vi "实时数据发送 (子VI).vi"(11 "数值":i32) -> ()   [LabVIEW 2016, in "数据传输系统.lvlib"]
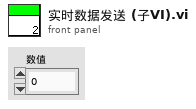
[diagram p1: front panel]
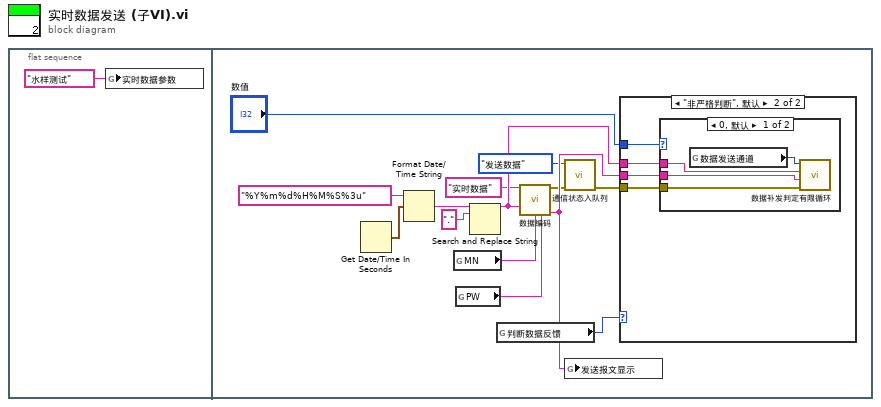
[diagram p0: block diagram]
diagram:
  n1 = flat-sequence {
    frame #0 {
      n2 = global write "全局 实时数据参数.vi" "实时数据参数"("水样测试" ("实时数据参数")) -> ()
    }
    frame #1 {
      n3 = Get Date/Time In Seconds() -> (seconds since 1Jan1904=w13:timestamp)
      n4 = Format Date/Time String(time format string (%c)="%Y%m%d%H%M%S%3u" ("时间格式字符串(%c)"), seconds (now)=w13) -> (date/time string=w12:string)  [unwired: 1 in]
      n5 = global read "断电保存全局.vi" "MN"() -> (w6:string)
      n6 = global read "断电保存全局.vi" "PW"() -> (w7:string)
      n7 = Search and Replace String(input string=w12, search string="." ("搜索字符串")) -> (result string=w15:string)  [unwired: 6 in, 3 out]
      n8 = global read "断电保存全局.vi" "判断数据反馈"() -> (w9:enum16{"非严格判断", "严格判断", "不判断"})
      n9 = call "数据编码.vi"("table输入"="实时数据" ("新元素/子数组"), "QN"=w15, "MN"=w6, "PW"=w7) -> ("错误常量"=w5:errorcluster, "通讯包字符串"=w10:string)  [unwired: 10 in]
      n10 = call "通信状态入队列.vi"("错误输入（无错误）"=w5, "枚举"=enum16{"打开连接", "发送数据", "读取数据", "数据处理", "关闭连接"}."发送数据") -> ("错误输出"=w8:errorcluster)  [unwired: 9 in]
      n11 = global write "全局1.vi" "发送报文显示"(w10) -> ()
      n12 = case shown="\"非严格判断\", 默认" w9 {
        tunnel: w10 -> [_ w19]
        tunnel: w8 -> [_ w18]
        tunnel: "数值" -> [_ w17]
        tunnel: w15 -> [_ w16]
        frame "不判断" {
        }
        frame "非严格判断", Default {
          n13 = case shown="0, 默认" w17 {
            tunnel: w19 -> [w23 _]
            tunnel: w18 -> [w22 _]
            tunnel: w16 -> [w20 _]
            frame 0, Default {
              n14 = global read "断电保存全局.vi" "数据发送通道"() -> (w21:enum16{"TCP", "VISA"})
              n15 = call "数据补发判定有限循环.vi"("错误输入（无错误）"=w22, "数据输入"=w23, "QN"=w20, "数据发送通道"=w21) -> ()  [unwired: 7 in, 1 out]
            }
            frame 14..17, 27..30 {
            }
          }
        }
      }
    }
  }
